vi "Populate Chan FPGA Data.vi"(6 "Channel descriptors in":T1, 8 "error in (no error)":errorcluster, 11 "FPGA Interface Base in":refnum<class "FPGA Interface Base.lvclass">) -> (0 "error out":errorcluster, 3 "FPGA Interface Base out":refnum<class "FPGA Interface Base.lvclass">, 4 "Channel descriptors out":T1)   [LabVIEW 2011, in "Engine Sim RT.lvlib"]
uses:
  Engine Sim RT.lvlib
  <userlib>/_FPGA Interface Advanced Tools/FPGA Interface Base/FPGA Interface Base.lvclass
  Shared/Channel Descriptors.ctl
  Shared/FPGA Write Descriptor.ctl
  Shared/InputChannelTypes.ctl
  <vilib>/rvi/DataTransferAndStorage/Container/Common/niFpgaDataTypeControl.ctl
  Shared/FPGA Read Descriptor.ctl
  Shared/OutputChannelTypes.ctl
  Shared/Status Chan Descriptor.ctl
  <userlib>/_FPGA Interface Advanced Tools/FPGA Interface Base/FPGA Interface Base.lvclass/FPGA Interface Base.ctl
  <vilib>/Utility/error.llb/Error Cluster From Error Code.vi
  Engine Simulation Shared.lvlib
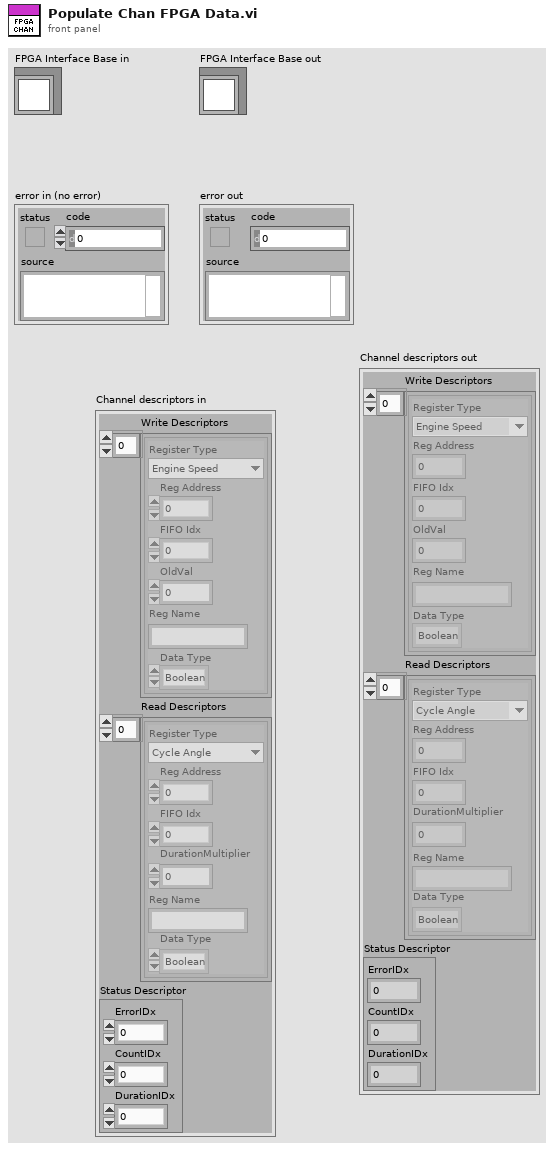
[diagram p1: front panel]
types:
  T1 = typedef "Engine Simulation Shared.lvlib/Channel Descriptors.ctl" = cluster{"Write Descriptors":T2[], "Read Descriptors":T5[], "Status Descriptor":T7}
  T2 = typedef "Engine Simulation Shared.lvlib/FPGA Write Descriptor.ctl" = cluster{"Register Type":T3, "Reg Address":u32, "FIFO Idx":i32, "OldVal":dbl, "Reg Name":string, "Data Type":T4}
  T3 = typedef "Engine Simulation Shared.lvlib/InputChannelTypes.ctl" = enum16{"Engine Speed", "Offset"}
  T4 = typedef "niFpgaDataTypeControl.ctl" = enum32{"Boolean", "I8", "I16", "I32", "I64", "U8", "U16", "U32", "U64", "FXP", "CustomControl"}
  T5 = typedef "Engine Simulation Shared.lvlib/FPGA Read Descriptor.ctl" = cluster{"Register Type":T6, "Reg Address":u32, "FIFO Idx":i32, "DurationMultiplier":dbl, "Reg Name":string, "Data Type":T4}
  T6 = typedef "Engine Simulation Shared.lvlib/OutputChannelTypes.ctl" = enum16{"Cycle Angle", "Crank Angle", "Time Duration", "Angle Duration", "Start Angle", "End Angle"}
  T7 = typedef "Engine Simulation Shared.lvlib/Status Chan Descriptor.ctl" = cluster{"ErrorIDx":i32, "CountIDx":i32, "DurationIDx":i32}
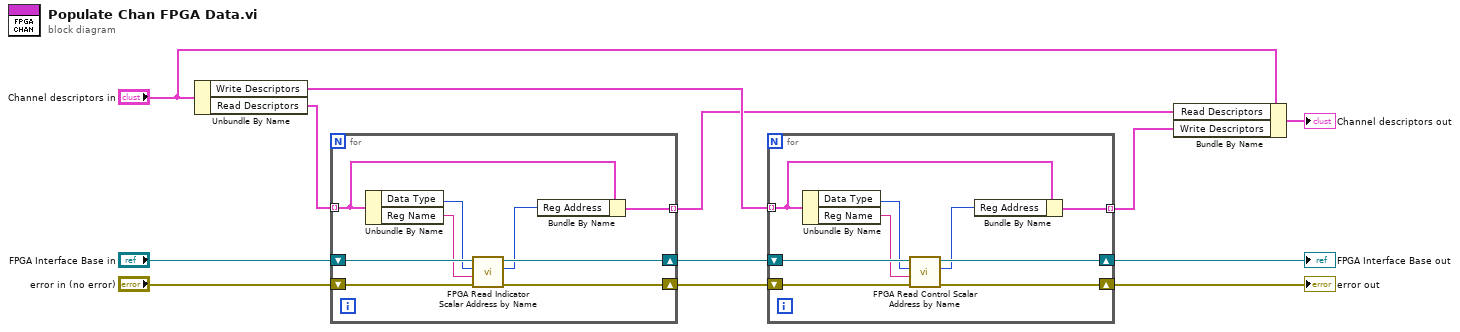
[diagram p0: block diagram]
diagram:
  n1 = Unbundle By Name("Channel descriptors in") -> ("Write Descriptors"=w7:T2[], "Read Descriptors"=w10:T5[])
  n2 = for {
    shift-right: [w19] -> w9
    shift-left: "error in (no error)" -> [w21]
    shift-right: [w18] -> w8
    shift-left: "FPGA Interface Base in" -> [w20]
    tunnel: w10 -> [w17] mode=indexing
    tunnel: [w15] -> w5 mode=indexing
    n3 = Unbundle By Name(w17) -> ("Data Type"=w14:T4, "Reg Name"=w13:string)
    n4 = call <userlib>:"FPGA Read Indicator Scalar Address by Name.vi"("error in (no error)"=w21, "Name"=w13, "Data Type"=w14, "FPGA Interface Base in"=w20) -> ("error out"=w19:errorcluster, "Address"=w16:u32, "FPGA Interface Base out"=w18:refnum<class "FPGA Interface Base.lvclass">)  [unwired: 4 in, 1 out]
    n5 = Bundle By Name(cluster=w17, "Reg Address"=w16) -> (w15:T5)
  }
  n6 = for {
    shift-right: [w28] -> w3
    shift-left: w9 -> [w30]
    shift-right: [w27] -> w2
    shift-left: w8 -> [w29]
    tunnel: w7 -> [w26] mode=indexing
    tunnel: [w24] -> w4 mode=indexing
    n7 = Unbundle By Name(w26) -> ("Data Type"=w23:T4, "Reg Name"=w22:string)
    n8 = call <userlib>:"FPGA Read Control Scalar Address by Name.vi"("error in (no error)"=w30, "Name"=w22, "Data Type"=w23, "FPGA Interface Base in"=w29) -> ("error out"=w28:errorcluster, "Address"=w25:u32, "FPGA Interface Base out"=w27:refnum<class "FPGA Interface Base.lvclass">)  [unwired: 4 in, 1 out]
    n9 = Bundle By Name(cluster=w26, "Reg Address"=w25) -> (w24:T2)
  }
  "FPGA Interface Base out" <- w2
  "error out" <- w3
  n10 = Bundle By Name(cluster="Channel descriptors in", "Read Descriptors"=w5, "Write Descriptors"=w4) -> (→"Channel descriptors out":T1)
